vi "get_quantity.vi"(7 "Quantity Name":string, 8 "error in":errorcluster) -> (0 "error out":errorcluster, 3 "Quantity Value":T1={"Name"="A", "Value"=[1.0], "Uncertainty"=[[1.0]], "Degrees of\nFreedom"=[10.0]})   [LabVIEW 2013]
uses:
  TD Quantity.ctl
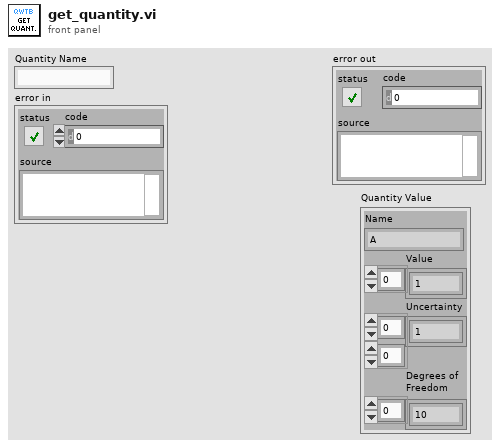
[diagram p1: front panel]
types:
  T1 = typedef "TD Quantity.ctl" = cluster{"Name":string, "Value":dbl[], "Uncertainty":dbl[][], "Degrees of\nFreedom":dbl[]}
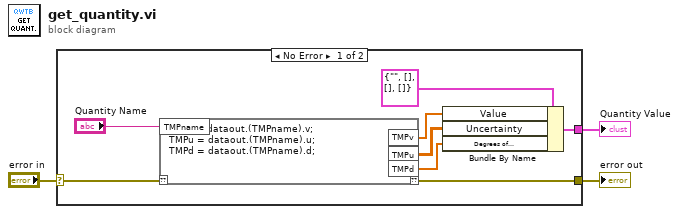
[diagram p0: block diagram]
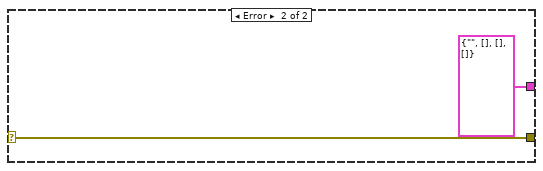
[diagram p2: hidden frame]
diagram:
  n1 = case shown="No Error" "error in" {
    selector: "error in" -> [w6 w13]
    tunnel: [w10 w13] -> w3
    tunnel: [w5 T1 {"Name"="", "Value"=[], "Uncertainty"=[], "Degrees of\nFreedom"=[]} ("Quantity")] -> w1
    frame No Error {
      n2 = script code="TMPv = dataout.(TMPname).v;\nTMPu = dataout.(TMPname).u;\nTMPd = dataout.(TMPname).d;"("??"=w6, "TMPname"="Quantity Name") -> ("??"=w10:errorcluster, "TMPv"=w8:dbl[], "TMPu"=w7:dbl[][], "TMPd"=w4:dbl[])
      n3 = Bundle By Name(cluster=T1 {"Name"="", "Value"=[], "Uncertainty"=[], "Degrees of\nFreedom"=[]} ("Quantity"), "Value"=w8, "Uncertainty"=w7, "Degrees of\nFreedom"=w4) -> (w5:T1)
    }
    frame Error {
    }
  }
  "error out" <- w3
  "Quantity Value" <- w1
